vi "create_CommPort.vi"(8 "error in (no error)":errorcluster) -> (0 "error out":errorcluster, 3 "pdbm_testsys_feedback_event":refnum<queue>)   [LabVIEW 2015, in "pdbm_test_system.lvlib"]
uses:
  pdbm_test_system.lvlib
  UsrDefine/pdbm_testsystem_feedback_data.ctl
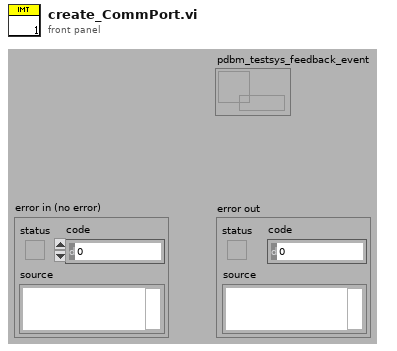
[diagram p1: front panel]
types:
  T1 = typedef "pdbm_test_system.lvlib/pdbm_testsystem_feedback_data.ctl" = cluster{"TaskName":string, "Request":string, "Data":variant}
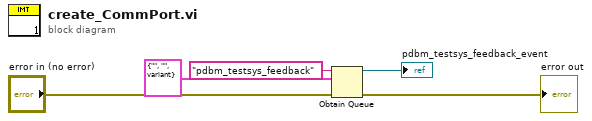
[diagram p0: block diagram]
diagram:
  n1 = Obtain Queue(name (unnamed)="pdbm_testsys_feedback", element data type=T1 {"TaskName"="", "Request"="", "Data"=variant} ("pdbm_test_system_feedback data"), error in (no error)="error in (no error)") -> (queue out=→"pdbm_testsys_feedback_event":refnum<queue>, error out=→"error out":errorcluster)  [unwired: 2 in, 1 out]
